vi "MoveAbsSingle.vi"(0 "controller in":refnum<k24>, 5 "axis name":string, 7 "speed":dbl, 9 "distance":dbl, 11 "error in (no error)":errorcluster, 12 "return immediately":bool) -> (4 "controller out":refnum<k24>, 15 "error out":errorcluster)   [LabVIEW 2016]
uses:
  C:/Program Files (x86)/Aerotech/Ensemble/LabVIEW/8.2/Bin/Aerotech.Ensemble.dll
  Bin/Aerotech.Ensemble.dll
  C:/Program Files (x86)/Aerotech/Ensemble/LabVIEW/8.2/Bin/Aerotech.Ensemble.LabVIEW.dll
  Bin/Aerotech.Ensemble.LabVIEW.dll
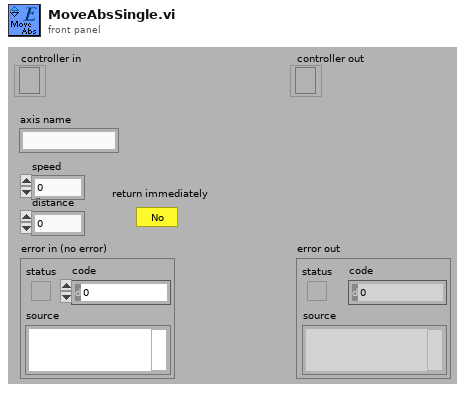
[diagram p1: front panel]
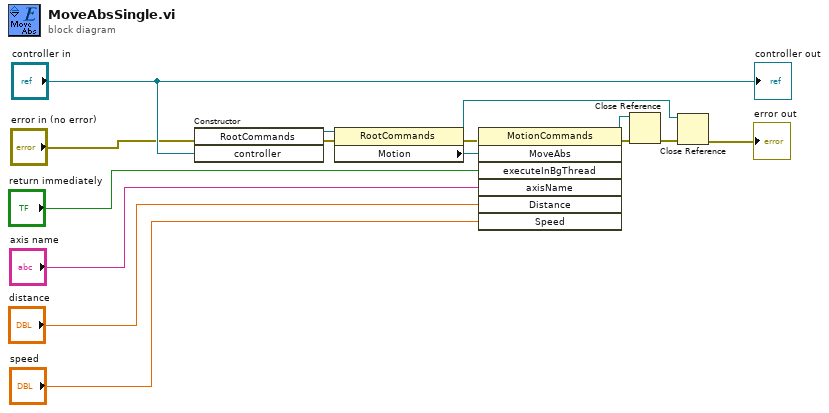
[diagram p0: block diagram]
diagram:
  n1 = constructor class="RootCommands"(error in="error in (no error)", "controller"="controller in") -> (reference out=w7:refnum<k24>, error out=w6:errorcluster)  [unwired: 2 in, 2 out]
  n2 = property class="RootCommands"(reference=w7, error in=w6) -> (reference out=w2:refnum<k24>, error out=w8:errorcluster, "Motion"=w9:refnum<k24>)
  n3 = invoke class="MotionCommands" method="MoveAbs"(reference=w9, error in=w8, "executeInBgThread"="return immediately", "axisName"="axis name", "Distance"="distance", "Speed"="speed") -> (reference out=w4:refnum<k24>, error out=w5:errorcluster)  [unwired: 1 in, 5 out]
  n4 = Close Reference(reference=w4, error in (no error)=w5) -> (error out=w3:errorcluster)
  n5 = Close Reference(reference=w2, error in (no error)=w3) -> (error out=→"error out":errorcluster)
  "controller out" <- "controller in"
